vi "Aux TE Controllers Close.vi"(8 "Error In":errorcluster, 11 "TE Serial Ports In":T1[](array[typedef]) {"XOFF Char" format="%.0x"; "XON Char" format="%.0x"; "flow control" items=["None"=0, "XON/XOFF"=1, "RTS/CTS"=2, "DTR/DSR"=4]; "stop bits" items=["1.0"=10, "1.5"=15, "2.0"=20]; "data bits" min=5 max=8 step=1; "baud rate" items=["75"=75, "110"=110, "134"=134, "150"=150, "300"=300, "600"=600, "1200"=1200, "1800"=1800, "2400"=2400, "4800"=4800, "7200"=7200, "9600"=9600, "14400"=14400, "19200"=19200, "28800"=28800, "38400"=38400, "56000"=56000, "57600"=57600, "115200"=115200, "128000"=128000, "230400"=230400]; "termination char" format="%.0x"}) -> (0 "Error Out":errorcluster, 1 "Regulators Off":bool, 3 "TE Serial Ports Out":T1[](array[typedef]) {"XOFF Char" format="%.0x"; "XON Char" format="%.0x"; "flow control" items=["None"=0, "XON/XOFF"=1, "RTS/CTS"=2, "DTR/DSR"=4]; "stop bits" items=["1.0"=10, "1.5"=15, "2.0"=20]; "data bits" min=5 max=8 step=1; "baud rate" items=["75"=75, "110"=110, "134"=134, "150"=150, "300"=300, "600"=600, "1200"=1200, "1800"=1800, "2400"=2400, "4800"=4800, "7200"=7200, "9600"=9600, "14400"=14400, "19200"=19200, "28800"=28800, "38400"=38400, "56000"=56000, "57600"=57600, "115200"=115200, "128000"=128000, "230400"=230400]; "termination char" format="%.0x"})   [LabVIEW 2016]
uses:
  Controls/Serial Visa Control.ctl
  Controls/SerialPortControl.ctl
panel:
  out "Loop active 2":bool
  out "Loop active":bool
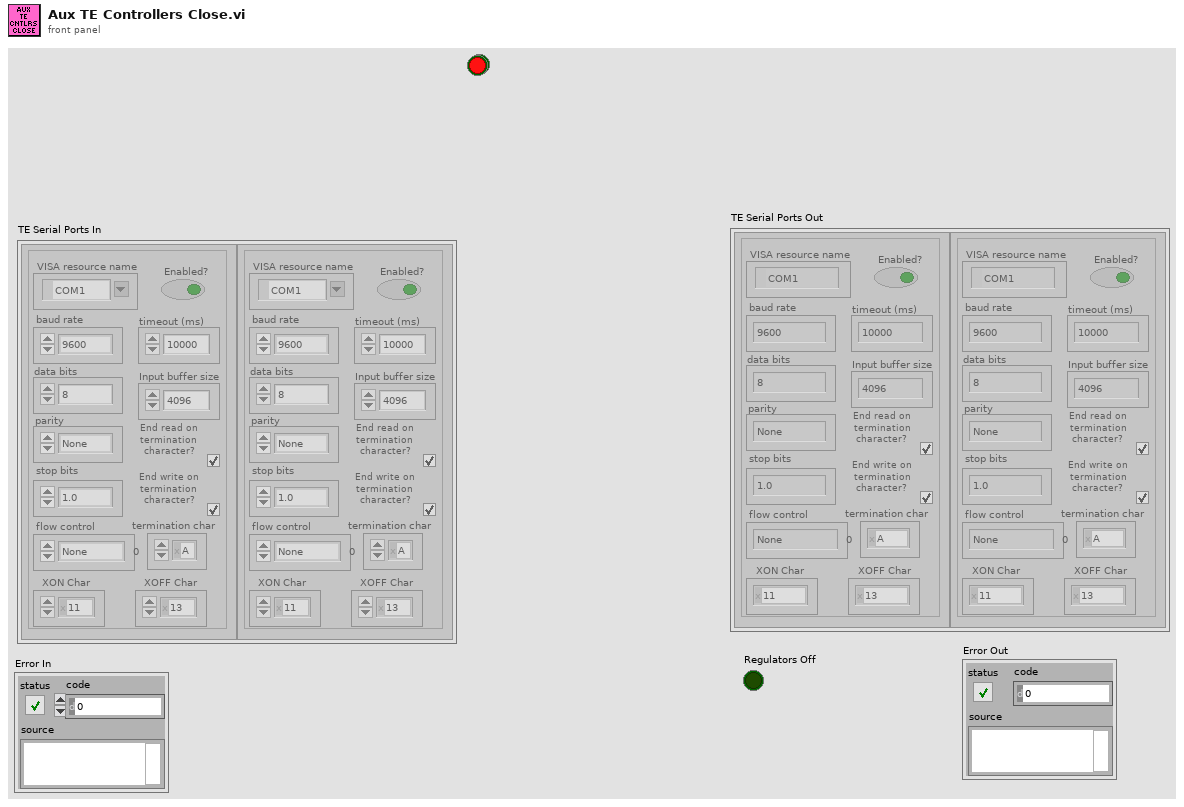
[diagram p1: front panel]
types:
  T1 = typedef "Serial Visa Control.ctl" = cluster{"termination char":u8, "End read on termination character?":bool, "Enabled?":bool, "VISA resource name":refnum<visa-resource-name>, "baud rate":u32, "data bits":u16, "parity":enum16{"None", "Odd", "Even", "Mark", "Space"}, "stop bits":u16, "flow control":u16, "timeout (ms)":u32, "Input buffer size":u32, "End write on termination character?":bool, "XON Char":u8, "XOFF Char":u8}
  T2 = typedef "SerialPortControl.ctl" = enum16{"Initialize", "Write Data", "Read Data", "Close Port"}
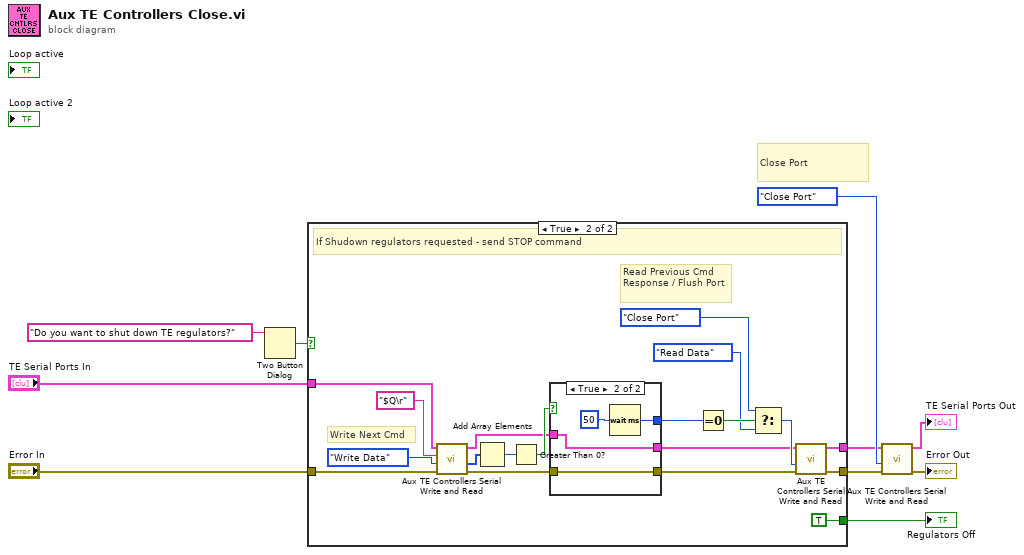
[diagram p0: block diagram]
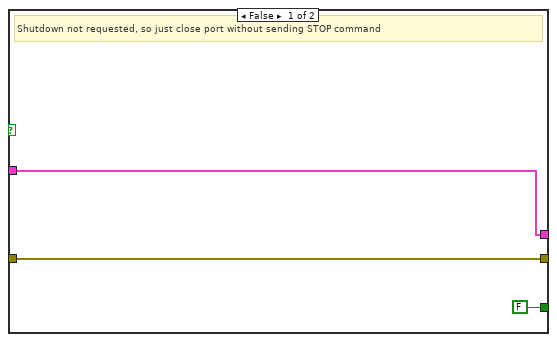
[diagram p2: hidden frame]
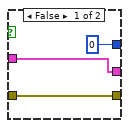
[diagram p3: hidden frame]
diagram:
  # "Close Port"
  n1 = Two Button Dialog(message="Do you want to shut down TE regulators?") -> (T button?=w1:bool)  [unwired: 2 in]
  n2 = case shown="True" w1 {
    tunnel: "Error In" -> [w12 w18]
    tunnel: "TE Serial Ports In" -> [w13 w17]
    tunnel: [w12 w16] -> w7
    tunnel: [w13 w15] -> w6
    tunnel: [FALSE TRUE] -> w3
    frame False {
      # "Shutdown not requested, so just close port without sending STOP command"
    }
    frame True {
      # "Read Previous Cmd Response / Flush Port"
      # "Write Next Cmd"
      # "If Shudown regulators requested - send STOP command"
      n3 = call "Aux TE Controllers Serial Write and Read.vi"("error in"=w18, "Action"=SerialPortControl."Write Data", "string to write"="$Q\r", "TE Controller Serial Ports In"=w17) -> ("Error Out"=w23:errorcluster, "#Bytes R/W"=w27:i16[], "TE Controller Serial Ports Out"=w21:T1[])  [unwired: 1 in, 2 out]
      n4 = Add Array Elements(numeric array=w27) -> (sum=w25:i16)
      n5 = Greater Than 0?(x=w25) -> (x > 0?=w26:bool)
      n6 = case shown="True" w26 {
        tunnel: [w34 w39] -> w22
        tunnel: w21 -> [w34 w39]
        tunnel: [w35 w38] -> w24
        tunnel: w23 -> [w35 w38]
        tunnel: [u32 0 ("millisecond timer value") w36] -> w28
        frame False {
        }
        frame True {
          n7 = Wait (ms)(milliseconds to wait=i16 50 ("y")) -> (millisecond timer value=w36:u32)
        }
      }
      n8 = Equal To 0?(x=w28) -> (x = 0?=w31:bool)
      n9 = Select(t=SerialPortControl."Close Port" ("Action"), s=w31, f=SerialPortControl."Read Data" ("Action")) -> (s? t:f=w29:T2)
      n10 = call "Aux TE Controllers Serial Write and Read.vi"("error in"=w24, "Action"=w29, "TE Controller Serial Ports In"=w22) -> ("Error Out"=w16:errorcluster, "TE Controller Serial Ports Out"=w15:T1[])  [unwired: 2 in, 3 out]
    }
  }
  "Regulators Off" <- w3
  n11 = call "Aux TE Controllers Serial Write and Read.vi"("error in"=w7, "Action"=SerialPortControl."Close Port", "TE Controller Serial Ports In"=w6) -> ("Error Out"=→"Error Out":errorcluster, "TE Controller Serial Ports Out"=→"TE Serial Ports Out":T1[])  [unwired: 2 in, 3 out]
